vi "Position change example.vi"() -> ()   [LabVIEW 2012]
panel:
  out "Position Change?":bool
  in  "Motor":i32=1 min=1 max=8 step=1
  in  "Position":dbl(slide) scale=0.0..200.0
  out "Output":dbl[](array[numeric])
  out "error out":errorcluster
  out "Position":dbl
  out "Index":i32
  in  "stop":bool
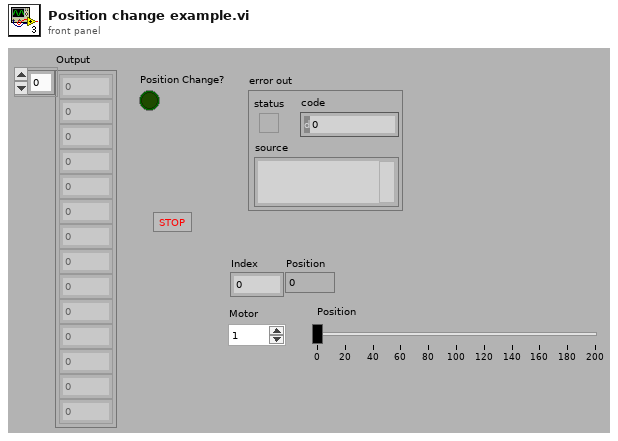
[diagram p1: front panel]
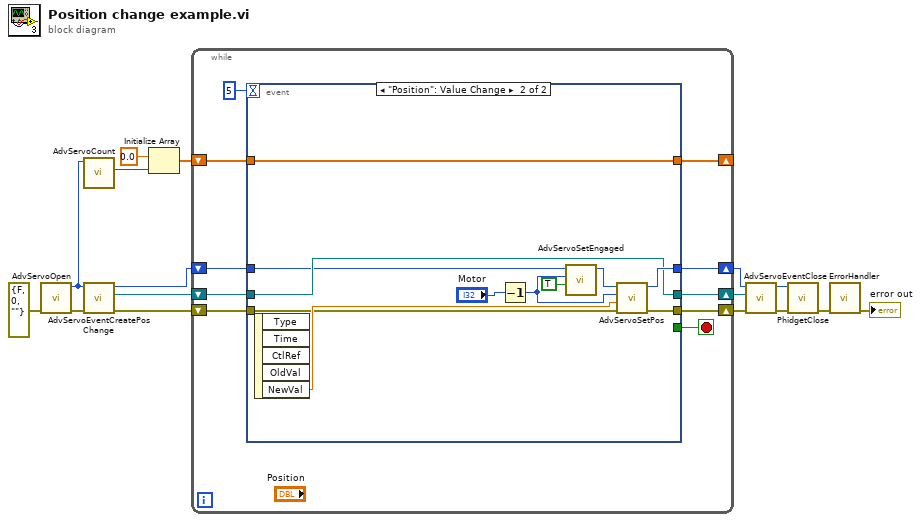
[diagram p0: block diagram]
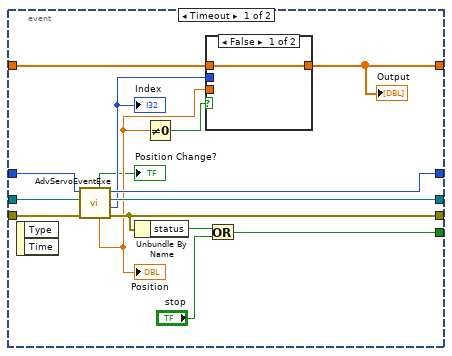
[diagram p2: hidden frame]
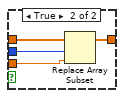
[diagram p3: hidden frame]
diagram:
  n1 = call "AdvServoOpen.vi"("error in"=errorcluster {"status"=FALSE, "code"=0, "source"=""}) -> ("error out"=w8:errorcluster, "Device Out"=w4:i32)  [unwired: 7 in, 2 out]
  n2 = call "AdvServoCount.vi"("Device In"=w4) -> ("count"=w2:i32)  [unwired: 8 in, 2 out]
  n3 = call "AdvServoEventCreatePosChange.vi"("error in (no error)"=w8, "Device In"=w4) -> ("error out"=w10:errorcluster, "Event Registration Refnum Out"=w12:refnum<event-registration>, "Device Out"=w14:i32)  [unwired: 7 in]
  n4 = Initialize Array(0.0 ("element"), w2) -> (w1:dbl[])
  n5 = while {
    shift-right: [w23] -> w11
    shift-left: w12 -> [w24]
    shift-right: [w25] -> w13
    shift-left: w14 -> [w26]
    shift-right: [w20] -> w7
    shift-left: w10 -> [w22]
    shift-right: [w18] -> _
    shift-left: w1 -> [w19]
    stop <- w21 stop-if-true
    n6 = event shown="[1] \"Position\": Value Change" {
      selector: _ -> [_ _]
      dyn-events: _ -> [_ _]
      timeout: 5 -> [_ _]
      tunnel: w26 -> [w41 w51]
      tunnel: [w40 w54] -> w25
      tunnel: w24 -> [w39 w53]
      tunnel: [w38 w53] -> w23
      tunnel: w22 -> [w37 w56]
      tunnel: [w35 _] -> w21
      tunnel: [w34 w55] -> w20
      tunnel: w19 -> [w32 w52]
      tunnel: [w30 w52] -> w18
      event Timeout {
        n7 = event-data() -> ()  [unwired: 1 in, 2 out]
        n8 = call "AdvServoEventExe.vi"("error in (no error)"=w37, "Event Registration Refnum In"=w39, "Device In"=w41) -> ("error out"=w34:errorcluster, "index"=w31:i32, "Event Registration Refnum Out"=w38:refnum<event-registration>, "Device Out"=w40:i32, "Value"=w29:dbl, "Event?"=→"Position Change?":bool)  [unwired: 3 in]
        "Index" <- w31
        "Position" <- w29
        n9 = Unbundle By Name(w34) -> ("status"=w33:bool)
        n10 = Not Equal To 0?(x=w29) -> (x != 0?=w28:bool)
        n11 = case shown="False" w28 {
          tunnel: w32 -> [w42 w46]
          tunnel: w31 -> [_ w45]
          tunnel: [w42 w44] -> w30
          tunnel: w29 -> [_ w43]
          frame False {
          }
          frame True {
            n12 = Replace Array Subset(array=w46, new element=w43, index=w45) -> (w44:dbl[])
          }
        }
        "Output" <- w30
        n13 = Or(x=w33, y="stop") -> (x .or. y?=w35:bool)
      }
      event "Position": Value Change {
        n14 = event-data() -> ("NewVal"=w57:dbl)  [unwired: 1 in, 4 out]
        n15 = Decrement(x="Motor") -> (x-1=w48:i32)
        n16 = call "AdvServoSetEngaged.vi"("SetEngaged"=TRUE, "index"=w48, "Device In"=w51) -> ("Device Out"=w50:i32)  [unwired: 6 in, 1 out]
        n17 = call "AdvServoSetPos.vi"("error in (no error)"=w56, "pos_in"=w57, "index"=w48, "Device In"=w50) -> ("error out"=w55:errorcluster, "Device Out"=w54:i32)  [unwired: 5 in]
      }
    }
  }
  n18 = call "AdvServoEventClose.vi"("error in (no error)"=w7, "Event Registration Refnum In"=w11, "Device In"=w13) -> ("error out"=w15:errorcluster, "Device Out"=w16:i32)  [unwired: 7 in]
  n19 = call "PhidgetClose.vi"("error in"=w15, "Device In"=w16) -> ("error out"=w6:errorcluster)  [unwired: 9 in]
  n20 = call "ErrorHandler.vi"("error in"=w6) -> ("error out"=→"error out":errorcluster)  [unwired: 9 in, 1 out]
